vi "Host Image Acquisition Loop.vi"(8 "error in":errorcluster) -> (0 "error out":errorcluster)   [LabVIEW 2013]
doc: "Loop handles the image acquisition communication to FPGA.\nInitialize - Queues up the intialize states\n\nExit"
uses:
  Host Image Acquisition Module Enum.ctl
  Message Passing/MsgQ Loops enum.ctl
  Image Acquisition Settings FG Enum.ctl
  System Status/Status FG Enum.ctl
  Globals/Simulation Settings Global.vi
  Common/State Machines/State Machine Lib.lvlib
  Message Passing/Main MsgQ.lvlib
panel:
  out "State":string
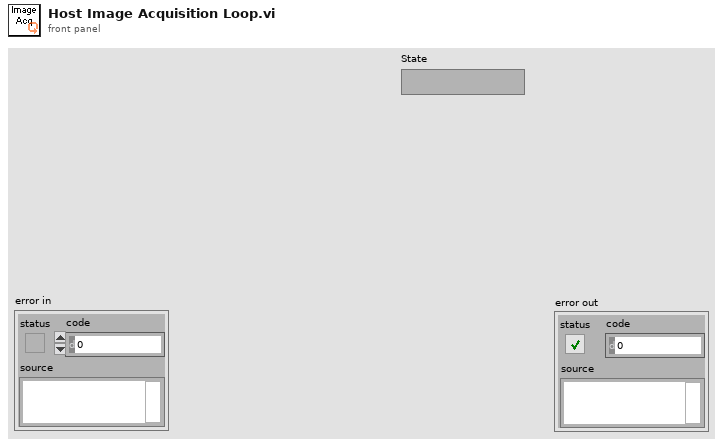
[diagram p1: front panel]
types:
  T1 = typedef "State Machine Lib.lvlib/STATE cluster.ctl" = cluster{"State":string, "Parameters":variant}
  T2 = typedef "Host Image Acquisition Module Enum.ctl" = enum16{"Open FPGA", "Initialize DMA FIFO", "Load Sim Images", "Initialize Acquisition", "Update Sector Parameters", "Start Acquisition", "Aquire Image", "Read Averages", "Cancel Acquisition", "Close FPGA"}
  T3 = typedef "Main MsgQ.lvlib/MsgQ Loops enum.ctl" = enum16{"User Interface", "Image Acq"}
  T4 = typedef "Image Acquisition Settings FG Enum.ctl" = enum16{"Read", "Write"}
  T5 = typedef "Status FG Enum.ctl" = enum16{"Reset", "Read", "Write"}
  T6 = typedef "Simulation Settings Cluster.ctl" = cluster{"Sim Enabled?":bool, "Sim Path":path}
  T7 = typedef "Acquisition Settings Cluster.ctl" = cluster{"Image Width":u32, "Image Height":u32, "Frames To Acquire":u32, "Signal Mapping":enum8{"Standard", "Basler 10-tap", "Vosskühler 10-tap"}, "DMA Buffer Size\n(In Images)":u32}
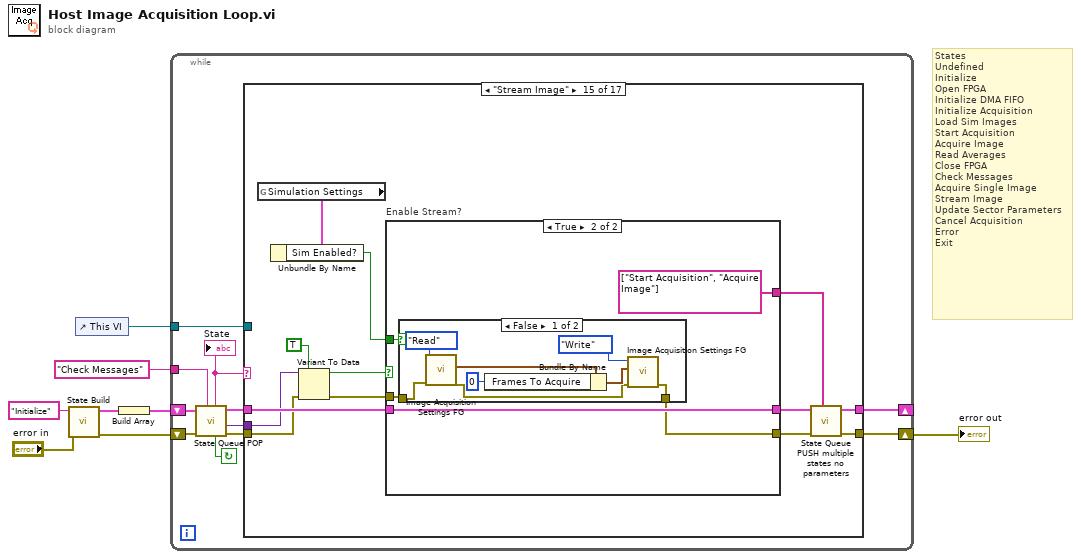
[diagram p0: block diagram]
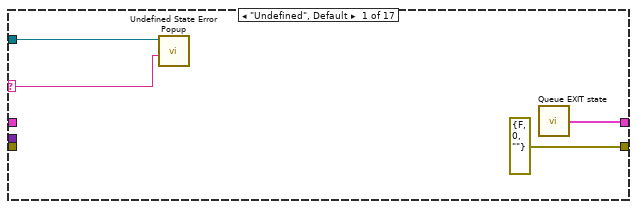
[diagram p2: hidden frame]
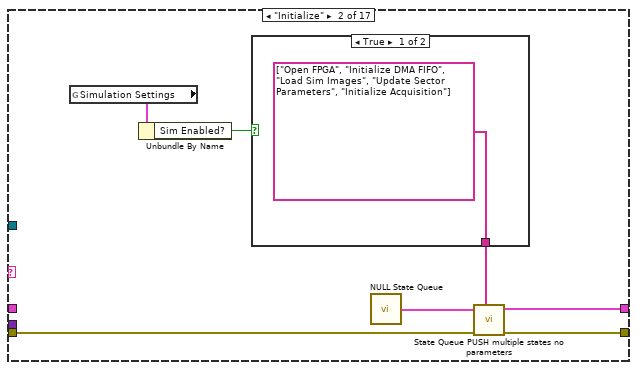
[diagram p3: hidden frame]
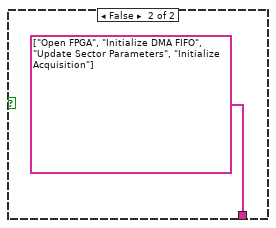
[diagram p4: hidden frame]
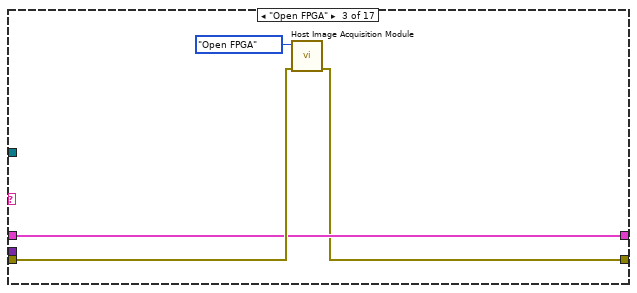
[diagram p5: hidden frame]
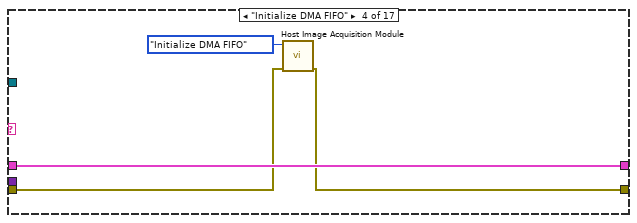
[diagram p6: hidden frame]
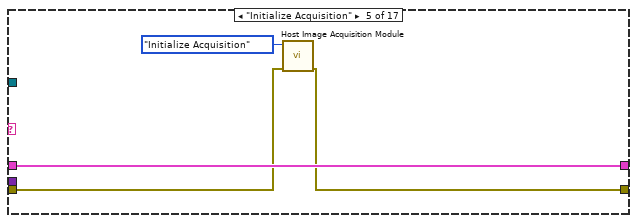
[diagram p7: hidden frame]
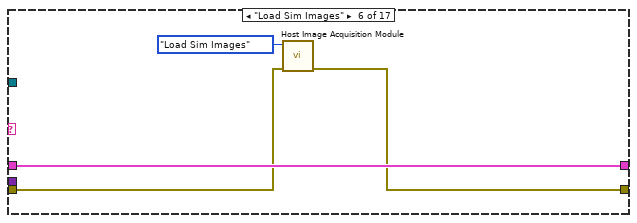
[diagram p8: hidden frame]
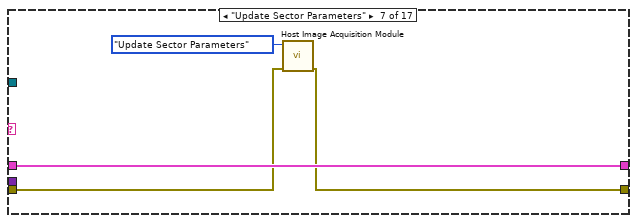
[diagram p9: hidden frame]
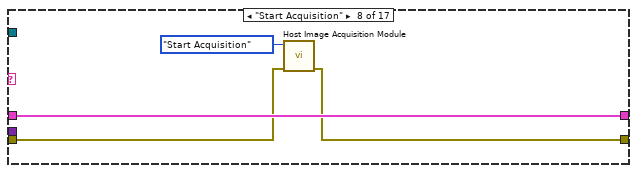
[diagram p10: hidden frame]
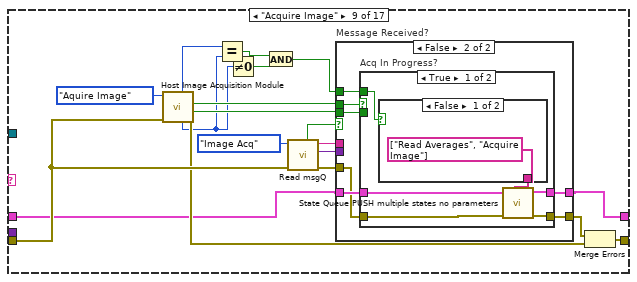
[diagram p11: hidden frame]
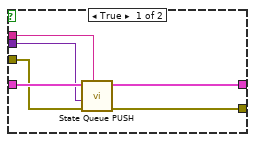
[diagram p12: hidden frame]
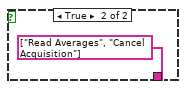
[diagram p13: hidden frame]
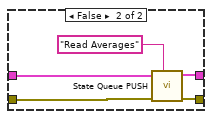
[diagram p14: hidden frame]
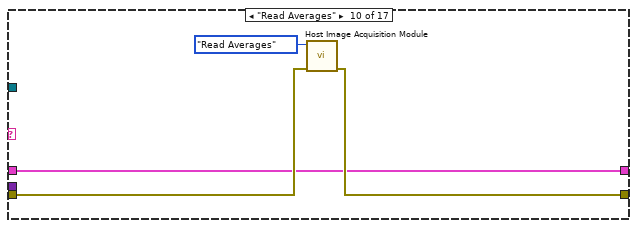
[diagram p15: hidden frame]
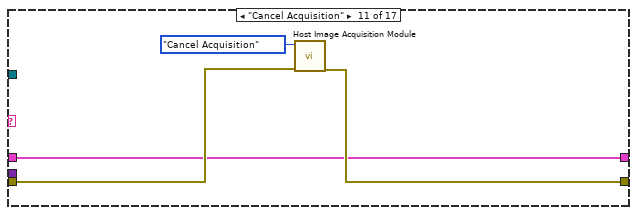
[diagram p16: hidden frame]
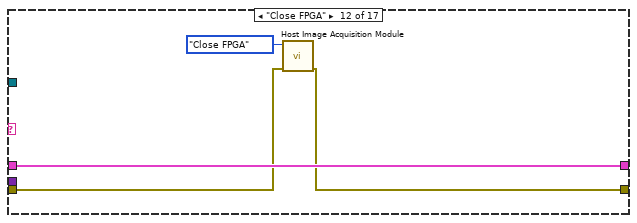
[diagram p17: hidden frame]
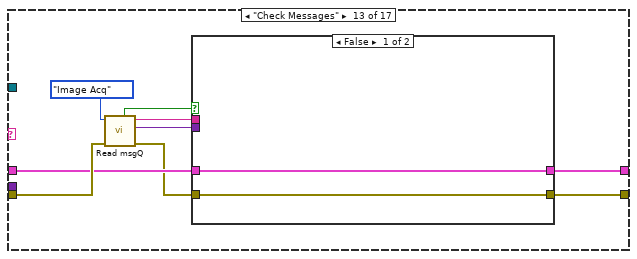
[diagram p18: hidden frame]
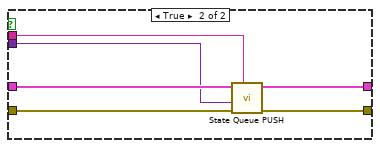
[diagram p19: hidden frame]
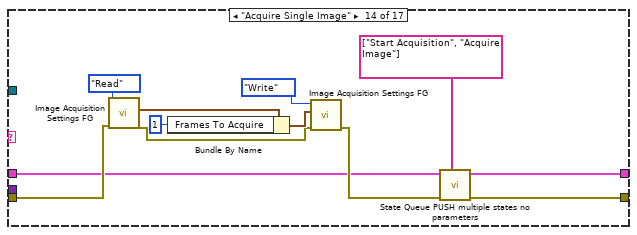
[diagram p20: hidden frame]
diagram:
  # "States\nUndefined\nInitialize\nOpen FPGA\nInitialize DMA FIFO\nInitialize Acquisition\nLoad Sim Images\nStart Acquisition\nAcquire Image\nRead Averages\nClose FPGA\nCheck Messages\nAcquire Single Image\nStream Image\nUpdate Sector Parameters\nCancel Acquisition\nError\nExit"
  n1 = call "State Build.vi"("error in (no error)"="error in", "State"="Initialize") -> ("error out"=w4:errorcluster, "State Out"=w6:T1)  [unwired: 8 in]
  n2 = control-ref of="This VI"() -> (w1:refnum<vi>)
  n3 = Build Array(w6) -> (w5:T1[])
  n4 = while {
    shift-right: [w12] -> _
    shift-left: w5 -> [w19]
    shift-right: [w11] -> w2
    shift-left: w4 -> [w18]
    tunnel: "Check Messages" ("Default state") -> [w16]
    tunnel: w1 -> [w10]
    stop <- w17 continue-if-true
    n5 = call "State Queue POP.vi"("Default state"=w16, "error in (no error)"=w18, "State que in"=w19) -> ("error out"=w13:errorcluster, "Parameters"=w9:variant, "State que out"=w14:T1[], "Not Exit?"=w17:bool, "State case out"=w15:string)  [unwired: 4 in]
    "State" <- w15
    n6 = case shown="\"Stream Image\"" w15 {
      selector: w15 -> [w22 _ _ _ _ _ _ _ _ _ _ _ _ _ _ _ _]
      tunnel: w14 -> [_ _ w34 w40 w44 w48 w52 w56 w67 w102 w106 w113 w120 w134 w155 w175 w182]
      tunnel: w13 -> [_ w30 w35 w39 w43 w47 w51 w55 w73 w104 w108 w112 w122 w141 w145 w178 w181]
      tunnel: [w21 w27 w34 w40 w44 w48 w52 w56 w65 w102 w106 w113 w119 w132 w150 w175 w182] -> w12
      tunnel: [errorcluster {"status"=FALSE, "code"=0, "source"=""} ("error out") w26 w33 w38 w42 w45 w50 w54 w71 w103 w107 w111 w118 w131 w148 w176 w181] -> w11
      tunnel: w10 -> [w23 _ _ _ _ _ _ _ _ _ _ _ _ _ _ _ _]
      tunnel: w9 -> [_ _ _ _ _ _ _ _ _ _ _ _ _ _ w154 _ _]
      frame "Undefined", Default {
        n7 = call "Undefined State Error Popup.vi"("String"=w22, "This VI (Caller if unwired)"=w23) -> ()  [unwired: 10 in]
        n8 = call "Queue EXIT state.vi"() -> ("Exit State Q"=w21:T1[])  [unwired: 1 in]
      }
      frame "Initialize" {
        n9 = global read "Simulation Settings Global.vi" "Simulation Settings"() -> (w25:T6)
        n10 = Unbundle By Name(w25) -> ("Sim Enabled?"=w24:bool)
        n11 = case shown="True" w24 {
          tunnel: [string[] ["Open FPGA", "Initialize DMA FIFO", "Load Sim Images", "Update Sector Parameters", "Initialize Acquisition"] ("States to queue") string[] ["Open FPGA", "Initialize DMA FIFO", "Update Sector Parameters", "Initialize Acquisition"] ("States to queue")] -> w28
          frame True {
          }
          frame False {
          }
        }
        n12 = call "NULL State Queue.vi"() -> ("NULL State Queue"=w29:T1[])
        n13 = call "State Queue PUSH multiple states no parameters.vi"("States to queue"=w28, "error in (no error)"=w30, "State que in"=w29) -> ("error out"=w26:errorcluster, "State que out"=w27:T1[])  [unwired: 7 in]
      }
      frame "Open FPGA" {
        n14 = call "Host Image Acquisition Module.vi"("error in"=w35, "Operation"=Host_Image_Acquisition_Module_Enum."Open FPGA") -> ("error out"=w33:errorcluster)  [unwired: 4 in, 5 out]
      }
      frame "Initialize DMA FIFO" {
        n15 = call "Host Image Acquisition Module.vi"("error in"=w39, "Operation"=Host_Image_Acquisition_Module_Enum."Initialize DMA FIFO") -> ("error out"=w38:errorcluster)  [unwired: 4 in, 5 out]
      }
      frame "Initialize Acquisition" {
        n16 = call "Host Image Acquisition Module.vi"("error in"=w43, "Operation"=Host_Image_Acquisition_Module_Enum."Initialize Acquisition") -> ("error out"=w42:errorcluster)  [unwired: 4 in, 5 out]
      }
      frame "Load Sim Images" {
        n17 = call "Host Image Acquisition Module.vi"("error in"=w47, "Operation"=Host_Image_Acquisition_Module_Enum."Load Sim Images") -> ("error out"=w45:errorcluster)  [unwired: 4 in, 5 out]
      }
      frame "Update Sector Parameters" {
        n18 = call "Host Image Acquisition Module.vi"("error in"=w51, "Operation"=Host_Image_Acquisition_Module_Enum."Update Sector Parameters") -> ("error out"=w50:errorcluster)  [unwired: 4 in, 5 out]
      }
      frame "Start Acquisition" {
        n19 = call "Host Image Acquisition Module.vi"("error in"=w55, "Operation"=Host_Image_Acquisition_Module_Enum."Start Acquisition") -> ("error out"=w54:errorcluster)  [unwired: 4 in, 5 out]
      }
      frame "Acquire Image" {
        n20 = call "Host Image Acquisition Module.vi"("error in"=w73, "Operation"=Host_Image_Acquisition_Module_Enum."Aquire Image") -> ("error out"=w72:errorcluster, "Image Acquired"=w63:bool, "Acq In Progress"=w64:bool, "Frames To Acquire"=w61:u32, "Num Frames read"=w68:u32)  [unwired: 4 in, 1 out]
        n21 = Equal?(x=w68, y=w61) -> (x = y?=w69:bool)
        n22 = Not Equal To 0?(x=w61) -> (x != 0?=w70:bool)
        n23 = And(x=w69, y=w70) -> (x .and. y?=w62:bool)
        n24 = call "Read msgQ.vi"("error in"=w73, "MsgQ enum"=MsgQ_Loops_enum."Image Acq") -> ("error out"=w57:errorcluster, "Message Received Parameters"=w58:variant, "Message Received String"=w59:string, "Message Recieved?"=w60:bool)  [unwired: 6 in]
        n25 = case "Message Received?" shown="False" w60 {
          tunnel: w67 -> [w81 w88]
          tunnel: [w80 w87] -> w66
          tunnel: [w79 w86] -> w65
          tunnel: w64 -> [_ w85]
          tunnel: w63 -> [_ w84]
          tunnel: w62 -> [_ w83]
          tunnel: w59 -> [w76 _]
          tunnel: w58 -> [w78 _]
          tunnel: w57 -> [w77 w82]
          frame True {
            n26 = call "State Queue PUSH.vi"("State case"=w76, "error in (no error)"=w77, "Parameters"=w78, "State que in"=w81) -> ("error out"=w80:errorcluster, "State que out"=w79:T1[])  [unwired: 6 in]
          }
          frame False {
            n27 = case "Acq In Progress?" shown="True" w85 {
              tunnel: w88 -> [w94 w101]
              tunnel: w82 -> [w91 w98]
              tunnel: [w92 w99] -> w87
              tunnel: [w93 w100] -> w86
              tunnel: w84 -> [_ _]
              tunnel: w83 -> [w89 _]
              frame True {
                n28 = case shown="False" w89 {
                  tunnel: [string[] ["Read Averages", "Acquire Image"] ("States to queue") string[] ["Read Averages", "Cancel Acquisition"] ("States to queue")] -> w90
                  frame False {
                  }
                  frame True {
                  }
                }
                n29 = call "State Queue PUSH multiple states no parameters.vi"("States to queue"=w90, "error in (no error)"=w91, "State que in"=w94) -> ("error out"=w92:errorcluster, "State que out"=w93:T1[])  [unwired: 7 in]
              }
              frame False {
                n30 = call "State Queue PUSH.vi"("State case"="Read Averages", "error in (no error)"=w98, "State que in"=w101) -> ("error out"=w99:errorcluster, "State que out"=w100:T1[])  [unwired: 7 in]
              }
            }
          }
        }
        n31 = Merge Errors(w66, w72) -> (w71:errorcluster)
      }
      frame "Read Averages" {
        n32 = call "Host Image Acquisition Module.vi"("error in"=w104, "Operation"=Host_Image_Acquisition_Module_Enum."Read Averages") -> ("error out"=w103:errorcluster)  [unwired: 4 in, 5 out]
      }
      frame "Cancel Acquisition" {
        n33 = call "Host Image Acquisition Module.vi"("error in"=w108, "Operation"=Host_Image_Acquisition_Module_Enum."Cancel Acquisition") -> ("error out"=w107:errorcluster)  [unwired: 4 in, 5 out]
      }
      frame "Close FPGA" {
        n34 = call "Host Image Acquisition Module.vi"("error in"=w112, "Operation"=Host_Image_Acquisition_Module_Enum."Close FPGA") -> ("error out"=w111:errorcluster)  [unwired: 4 in, 5 out]
      }
      frame "Check Messages" {
        n35 = call "Read msgQ.vi"("error in"=w122, "MsgQ enum"=MsgQ_Loops_enum."Image Acq") -> ("error out"=w117:errorcluster, "Message Received Parameters"=w114:variant, "Message Received String"=w116:string, "Message Recieved?"=w121:bool)  [unwired: 6 in]
        n36 = case shown="False" w121 {
          tunnel: w120 -> [w124 w130]
          tunnel: [w124 w129] -> w119
          tunnel: [w123 w128] -> w118
          tunnel: w117 -> [w123 w127]
          tunnel: w116 -> [_ w125]
          tunnel: w114 -> [_ w126]
          frame False {
          }
          frame True {
            n37 = call "State Queue PUSH.vi"("State case"=w125, "error in (no error)"=w127, "Parameters"=w126, "State que in"=w130) -> ("error out"=w128:errorcluster, "State que out"=w129:T1[])  [unwired: 6 in]
          }
        }
      }
      frame "Acquire Single Image" {
        n38 = call "Image Acquisition Settings FG.vi"("error in (no error)"=w141, "Operation"=Image_Acquisition_Settings_FG_Enum."Read") -> ("error out"=w136:errorcluster, "Acquisition Settings Out"=w140:T7)  [unwired: 8 in]
        n39 = Bundle By Name(cluster=w140, "Frames To Acquire"=u32 1) -> (w138:T7)
        n40 = call "Image Acquisition Settings FG.vi"("error in (no error)"=w136, "Acquisition Settings In"=w138, "Operation"=Image_Acquisition_Settings_FG_Enum."Write") -> ("error out"=w135:errorcluster)  [unwired: 7 in, 1 out]
        n41 = call "State Queue PUSH multiple states no parameters.vi"("States to queue"=string[] ["Start Acquisition", "Acquire Image"], "error in (no error)"=w135, "State que in"=w134) -> ("error out"=w131:errorcluster, "State que out"=w132:T1[])  [unwired: 7 in]
      }
      frame "Stream Image" {
        n42 = global read "Simulation Settings Global.vi" "Simulation Settings"() -> (w146:T6)
        n43 = Unbundle By Name(w146) -> ("Sim Enabled?"=w143:bool)
        n44 = Variant To Data(error in=w145, type=TRUE, Variant=w154) -> (data=w152:bool, error out=w144:errorcluster)
        n45 = case "Enable Stream?" shown="True" w152 {
          tunnel: w144 -> [w156 w163]
          tunnel: w155 -> [w157 w162]
          tunnel: [w157 w162] -> w151
          tunnel: [w156 w161] -> w149
          tunnel: [string[] ["Cancel Acquisition"] ("States to queue") string[] ["Start Acquisition", "Acquire Image"] ("States to queue")] -> w147
          tunnel: w143 -> [_ w159]
          frame False {
          }
          frame True {
            n46 = case shown="False" w159 {
              tunnel: w163 -> [w170 w172]
              tunnel: [w164 w172] -> w161
              frame False {
                n47 = call "Image Acquisition Settings FG.vi"("error in (no error)"=w170, "Operation"=Image_Acquisition_Settings_FG_Enum."Read") -> ("error out"=w165:errorcluster, "Acquisition Settings Out"=w169:T7)  [unwired: 8 in]
                n48 = Bundle By Name(cluster=w169, "Frames To Acquire"=u32 0) -> (w167:T7)
                n49 = call "Image Acquisition Settings FG.vi"("error in (no error)"=w165, "Acquisition Settings In"=w167, "Operation"=Image_Acquisition_Settings_FG_Enum."Write") -> ("error out"=w164:errorcluster)  [unwired: 7 in, 1 out]
              }
              frame True {
              }
            }
          }
        }
        n50 = call "State Queue PUSH multiple states no parameters.vi"("States to queue"=w147, "error in (no error)"=w149, "State que in"=w151) -> ("error out"=w148:errorcluster, "State que out"=w150:T1[])  [unwired: 7 in]
      }
      frame "Error" {
        n51 = Unbundle By Name(w178) -> ("source"=w179:string)
        n52 = Concatenate Strings("Error: " ("string"), w179) -> (w174:string)
        n53 = call "Status FG.vi"("Status In"=w174, "Operation"=Status_FG_Enum."Write") -> ()  [unwired: 8 in, 2 out]
        n54 = call "Broadcast Exit.vi"("error in"=errorcluster {"status"=FALSE, "code"=0, "source"=""}) -> ("error out"=w176:errorcluster)  [unwired: 10 in]
      }
      frame "Exit" {
      }
    }
  }
  "error out" <- w2
